vi "SetWindowText.vi"(8 "error in (no error)":errorcluster, 10 "window text (\"\")":string, 11 "hWnd (NULL)":T1) -> (0 "error out":errorcluster, 3 "dup hWnd":T1)   [LabVIEW 2011]
doc: "SetWindowText\nThe SetWindowText function changes the text of the specified window's title bar (if it has one). If the specified window is a control, the text of the control is changed. However, SetWindowText cannot change the text of a control in another application.\n\nBOOL SetWindowText(\n HWND hWnd, // handle to window or control\n LPCTSTR lpString // address of string\n);\n \nParameters\nhWnd \nHandle to the window or control whose text is to be changed. \nlpString \nPointer to a null-terminated string to be used as the new title or control text. \nReturn Values\nIf the function succeeds, the return value is nonzero.\n\nIf the function fails, the return value is zero. To get extended error information, callGetLastError. \n\nRemarks\nIf the target window is owned by the current process, SetWindowText causes a WM_SETTEXT message to be sent to the specified window or control. If the control is a list box control created with the WS_CAPTION style, however, SetWindowText sets the text for the control, not for the list box entries. \n\nThe SetWindowText function does not expand tab characters (ASCII code 0x09). Tab characters are displayed as vertical bar (|) characters."
uses:
  hWnd.ctl
  user32.dll
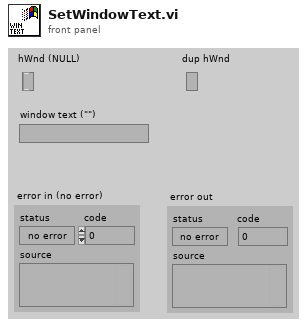
[diagram p1: front panel]
types:
  T1 = typedef "hWnd.ctl" = refnum<k1>
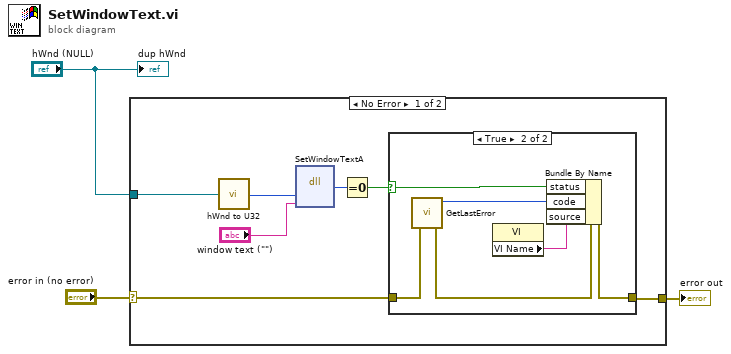
[diagram p0: block diagram]
diagram:
  n1 = case shown="No Error" "error in (no error)" {
    selector: "error in (no error)" -> [w4 w18]
    tunnel: [w6 w18] -> w3
    tunnel: "hWnd (NULL)" -> [w8 _]
    frame No Error {
      n2 = call "hWnd to U32.vi"("hWnd"=w8) -> ("hWnd"=w9:u32)  [unwired: 4 out]
      n3 = dll-call lib="User32.dll" fn="SetWindowTextA" label="SetWindowText"("hWnd"=w9, "lpString"="window text (\"\")") -> ("error"=w7:i32)  [unwired: 5 in, 2 out]
      n4 = Equal To 0?(x=w7) -> (x = 0?=w5:bool)
      n5 = case shown="True" w5 {
        selector: w5 -> [_ w12]
        tunnel: w4 -> [w11 w16]
        tunnel: [w11 w17] -> w6
        frame False {
        }
        frame True {
          n6 = call "GetLastError.vi"("error in (no error)"=w16) -> ("error out"=w15:errorcluster, "CODE"=w14:i32)  [unwired: 5 out]
          n7 = property class="VI"() -> ("VI Name"=w13:string)  [unwired: 2 in, 2 out]
          n8 = Bundle By Name(cluster=w15, "status"=w12, "code"=w14, "source"=w13) -> (w17:errorcluster)
        }
      }
    }
    frame Error {
    }
  }
  "error out" <- w3
  "dup hWnd" <- "hWnd (NULL)"
